vi "Setup subWorker - Maes-Acq.vi"(8 "error in":errorcluster, 11 "Maestro Control in":refnum<class "Maestro Control.lvclass">) -> (0 "error out":errorcluster, 3 "Maestro Control out":refnum<class "Maestro Control.lvclass">)   [LabVIEW 2021, in "Maestro Control.lvclass"]
doc: "<b>Note: Do not change the code in this VI!</b>\nThis VI performs a setup of all the statically-linked subWorkers that belong to the Worker that calls this VI. This VI is created automatically by the 'Create/Add Worker' tool and must be called <b>before</b> any statically linked subWorkers are called."
uses:
  Maestro Control.lvclass
  Maestro Control.lvclass/Maestro Control.ctl
  Maestro Acq/Maestro Acq.lvclass
  C:/Program Files (x86)/National Instruments/LabVIEW 2021/vi.lib/addons/_Workers/Library/Classes/Worker/Worker.lvclass
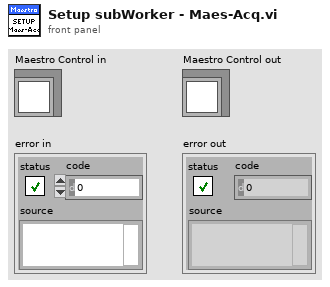
[diagram p1: front panel]
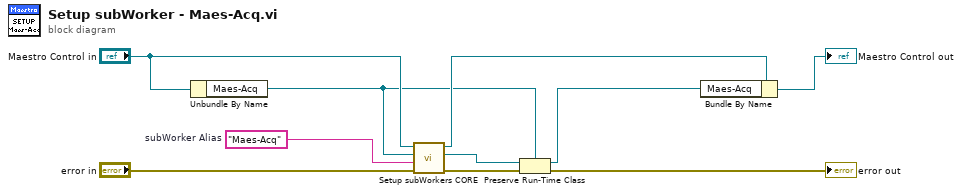
[diagram p0: block diagram]
diagram:
  w6 = "Maes-Acq"  # subWorker Alias
  n1 = Unbundle By Name("Maestro Control in") -> ("Maes-Acq"=w3:refnum<class "Maestro Acq.lvclass">)
  n2 = call-dynamic "Setup subWorkers CORE.vi"("error in"="error in", "subWorker Alias"=w6, "subWorker"=w3, "Worker"="Maestro Control in") -> ("error out"=w5:errorcluster, "subWorker out"=w1:refnum<class "Worker.lvclass">, "Worker out"=w8:refnum<class "Maestro Control.lvclass">)  [unwired: 5 in]
  n3 = Preserve Run-Time Class(object in=w1, error in=w5, 2:w3) -> (object out=w2:refnum<class "Maestro Acq.lvclass">, error out=→"error out":errorcluster)
  n4 = Bundle By Name(cluster=w8, "Maes-Acq"=w2) -> (→"Maestro Control out":refnum<class "Maestro Control.lvclass">)
